vi "Add Tool.vi"(8 "error in (no error)":errorcluster, 10 "tool":refnum<class "PyTool.lvclass">, 11 "PyServer in":refnum<class "PyServer.lvclass">) -> (0 "error out":errorcluster, 3 "PyServer out":refnum<class "PyServer.lvclass">)   [LabVIEW 2025, in "Tools.lvlib" / "PyServer.lvclass"]
uses:
  PyServer.lvclass
  PyServer.lvclass/PyServer.ctl
  PyTool/PyTool.lvclass
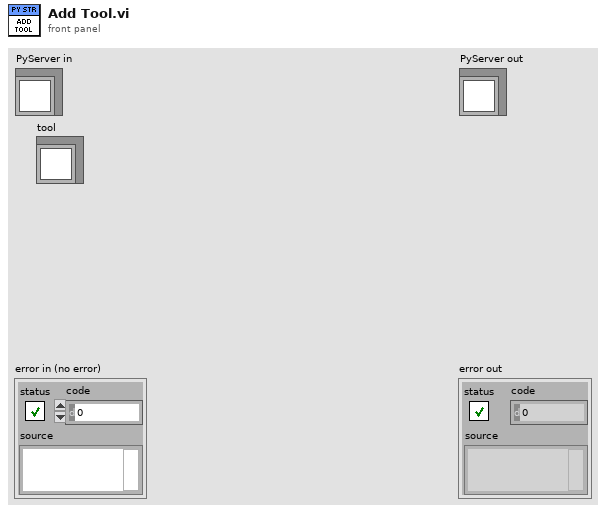
[diagram p1: front panel]
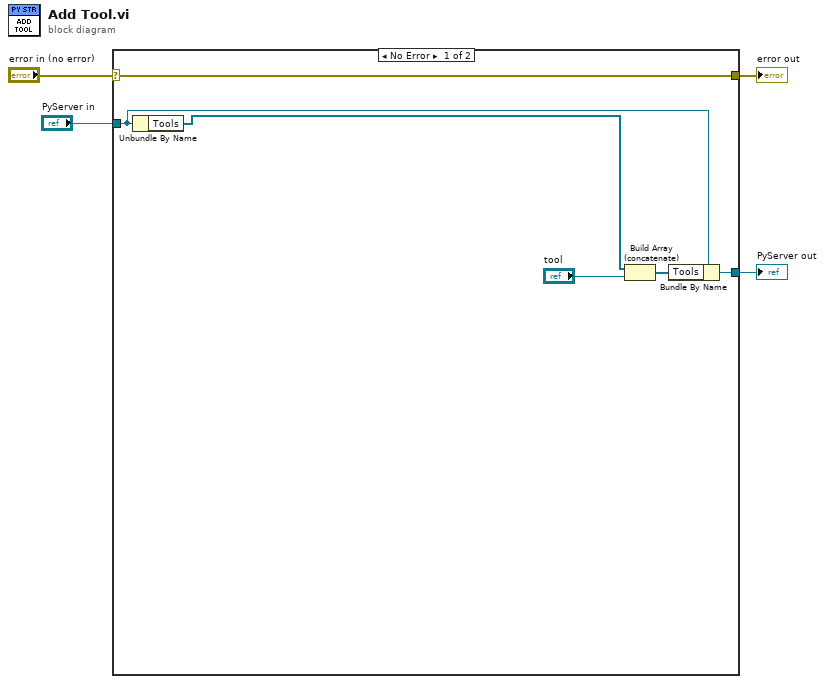
[diagram p0: block diagram]
diagram:
  n1 = case shown="No Error" "error in (no error)" {
    selector: "error in (no error)" -> [w10 w12]
    tunnel: [w10 w12] -> w3
    tunnel: [w9 w11] -> w1
    tunnel: "PyServer in" -> [w8 w11]
    frame No Error {
      n2 = Unbundle By Name(w8) -> ("Tools"=w7:refnum<class "PyTool.lvclass">[])
      n3 = Build Array (concatenate)(w7, "tool") -> (w6:refnum<class "PyTool.lvclass">[])
      n4 = Bundle By Name(cluster=w8, "Tools"=w6) -> (w9:refnum<class "PyServer.lvclass">)
    }
    frame Error {
    }
  }
  "error out" <- w3
  "PyServer out" <- w1
